vi "重采样.vi"(10 "重采样间隔":dbl, 11 "输出簇":cluster{"时间":dbl[], "力":dbl[]}) -> (3 "簇":cluster{"xi used":dbl[], "yi":dbl[]})   [LabVIEW 2019]
uses:
  <vilib>/gmath/NI_Gmath.lvlib
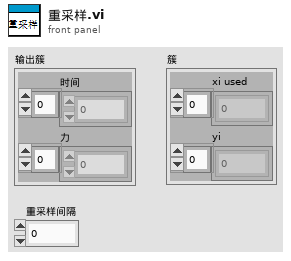
[diagram p1: front panel]
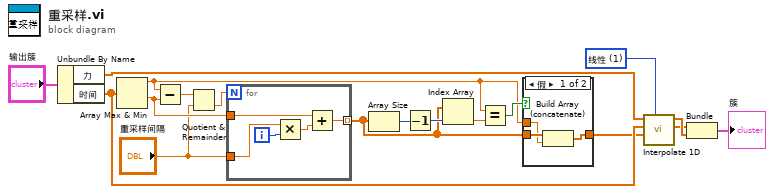
[diagram p0: block diagram]
diagram:
  w8 = 1 items=["最近", "线性", "样条", "cubic Hermite", "拉格朗日"] ("method")
  n1 = Unbundle By Name("输出簇") -> ("力"=w9:dbl[], "时间"=w10:dbl[])
  n2 = Array Max & Min(array=w10) -> (max value=w2:dbl, min value=w18:dbl)  [unwired: 2 out]
  n3 = Subtract(x=w2, y=w18) -> (x-y=w17:dbl)
  n4 = Quotient & Remainder(x=w17, y="重采样间隔") -> (floor(x/y)=w15:dbl)  [unwired: 1 out]
  n5 = for {
    N: w15 -> [_]
    tunnel: "重采样间隔" -> [w22]
    tunnel: w18 -> [w20]
    tunnel: [w19] -> w3 mode=indexing
    i -> [w23]
    n6 = Multiply(x=w22, y=w23) -> (x*y=w21:dbl)
    n7 = Add(x=w20, y=w21) -> (x+y=w19:dbl)
  }
  n8 = Array Size(array=w3) -> (size(s)=w6:i32)
  n9 = Decrement(x=w6) -> (x-1=w7:i32)
  n10 = Index Array(array=w3, index=w7) -> (element=w5:dbl)
  n11 = Equal?(x=w2, y=w5) -> (x = y?=w4:bool)
  n12 = case shown="假" w4 {
    tunnel: w3 -> [w26 w27]
    tunnel: w2 -> [w25 _]
    tunnel: [w24 w27] -> w1
    frame False {
      n13 = Build Array (concatenate)(w26, w25) -> (w24:dbl[])
    }
    frame True {
    }
  }
  n14 = call <vilib>:"Interpolate 1D.vi"("method"=w8, "xi"=w1, "X"=w10, "Y"=w9) -> ("xi used"=w11:dbl[], "yi"=w12:dbl[])  [unwired: 5 in, 1 out]
  n15 = Bundle("xi used"=w11, "yi"=w12) -> (→"簇":cluster{"xi used":dbl[], "yi":dbl[]})  [unwired: 1 in]
